vi "Filter Event Data.vi"(8 "error in (no error)":errorcluster, 10 "EventFilter Reference":T1, 11 "ControlDropMsg In":refnum<class "ControlDropMsg.lvclass">) -> (0 "error out":errorcluster, 2 "Discard?":bool, 3 "ControlDropMsg Out":refnum<class "ControlDropMsg.lvclass">)   [LabVIEW 2017, in "ActorEvents.lvlib" / "ControlDropMsg.lvclass"]
uses:
  ControlDropMsg.lvclass
  IEventFilter/EventFilter Reference.ctl
  IEventFilter/IEventFilter.lvclass
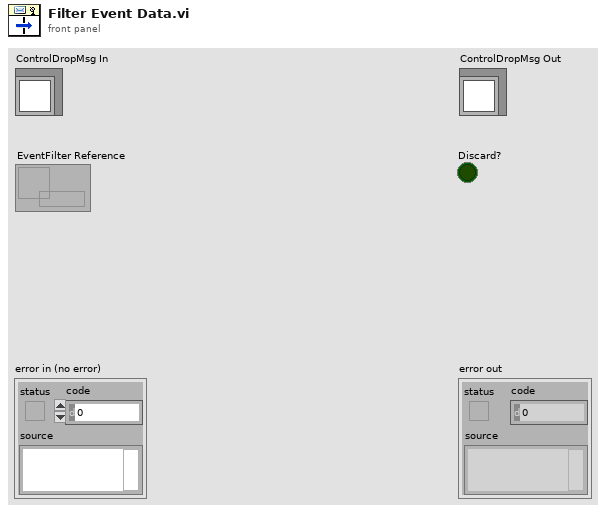
[diagram p1: front panel]
types:
  T1 = typedef "ActorEvents.lvlib/IEventFilter.lvclass/EventFilter Reference.ctl" = refnum<data-value>
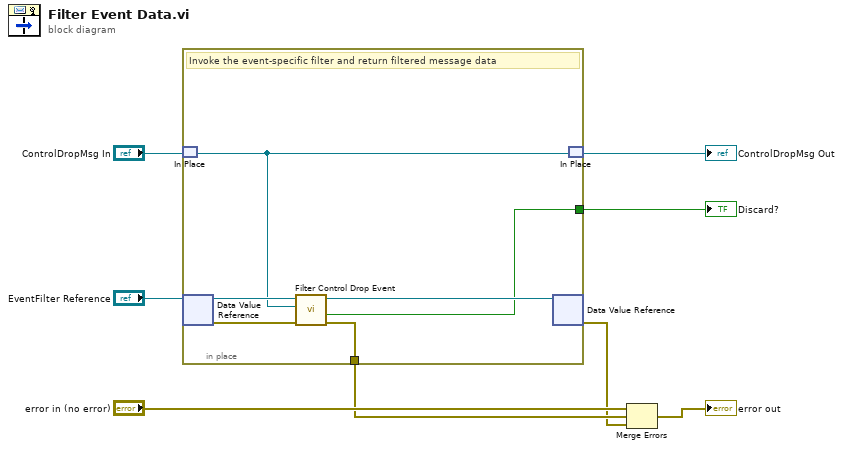
[diagram p0: block diagram]
diagram:
  n1 = in-place {
    in-place-border: [w10] -> w5
    in-place-border: [w11] -> w3
    # "Invoke the event-specific filter and return filtered message data"
    n2 = in-place-match #1("ControlDropMsg In") -> (w9:refnum<class "ControlDropMsg.lvclass">)
    n3 = in-place-dvr #2("EventFilter Reference") -> (w14:refnum<class "IEventFilter.lvclass">, w12:errorcluster)
    n4 = call-dynamic "Filter Control Drop Event.vi"("error in (no error)"=w12, "ControlDropMsg"=w9, "IEventFilter in"=w14) -> ("error out"=w10:errorcluster, "Discard?"=w11:bool, "IEventFilter out"=w13:refnum<class "IEventFilter.lvclass">)  [unwired: 6 in]
    n5 = in-place-dvr #2(w13) -> (w4:errorcluster)  [unwired: 1 out]
    n6 = in-place-match #1(w9) -> (→"ControlDropMsg Out":refnum<class "ControlDropMsg.lvclass">)
  }
  "Discard?" <- w3
  n7 = Merge Errors("error in (no error)", w5, w4) -> (→"error out":errorcluster)
